vi "LSCE1.vi"(0 "时间间隔":dbl format="%#_13g", 3 "数值输入控件":i32, 4 "相关函数":cluster{"f0":dbl, "df":dbl, "magnitude":dbl[]}(graph), 5 "FRF Phase":cluster{"f0":dbl, "df":dbl, "magnitude":dbl[]}(graph), 6 "FRF magnifitude":cluster{"f0":dbl, "df":dbl, "magnitude":dbl[]}(graph)) -> (1 "模态阻尼比":dbl[](array[numeric]), 2 "模态频率":dbl[](array[numeric]))   [LabVIEW 2014]
uses:
  <vilib>/Analysis/2dsp.llb/Inverse Real FFT.vi
  <vilib>/Analysis/baseanly.llb/Real A x B.vi
  <vilib>/Analysis/baseanly.llb/A x Vector.vi
  <vilib>/Analysis/baseanly.llb/Real Inverse Matrix.vi
  <vilib>/Analysis/polynomials.llb/Polynomial Roots (DBL).vi
  <vilib>/Analysis/NI_AALPro.lvlib
  <vilib>/Analysis/NI_AALBase.lvlib
panel:
  in  "error out":errorcluster caption="错误输出"
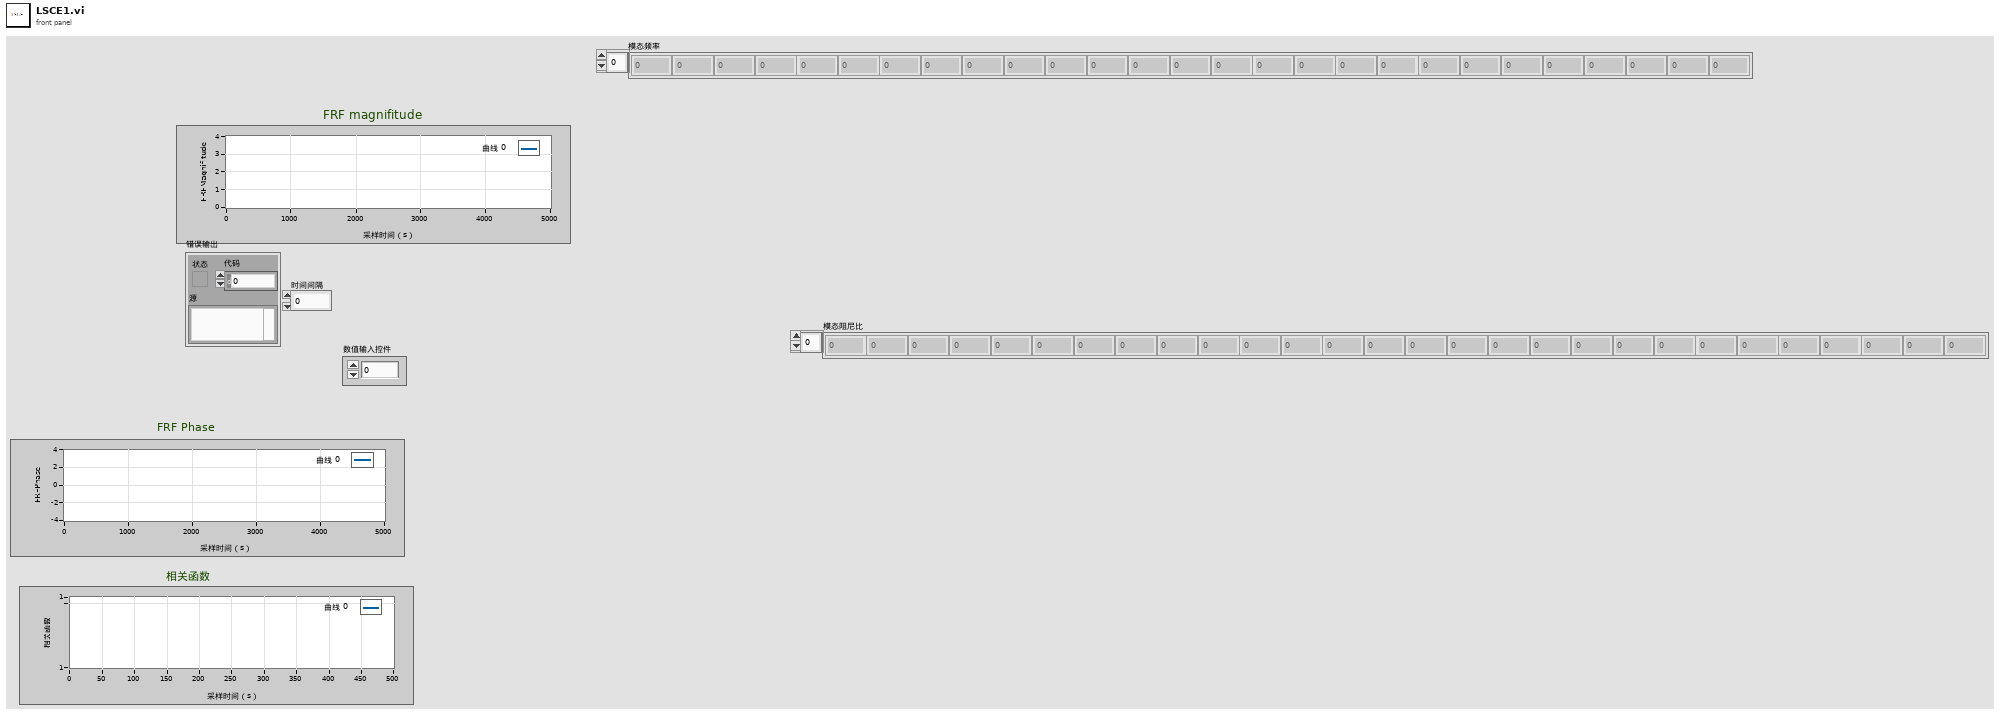
[diagram p1: front panel]
types:
  T1 = typedef "NI_Matrix.lvlib/RealMatrix.ctl" = dbl[][]
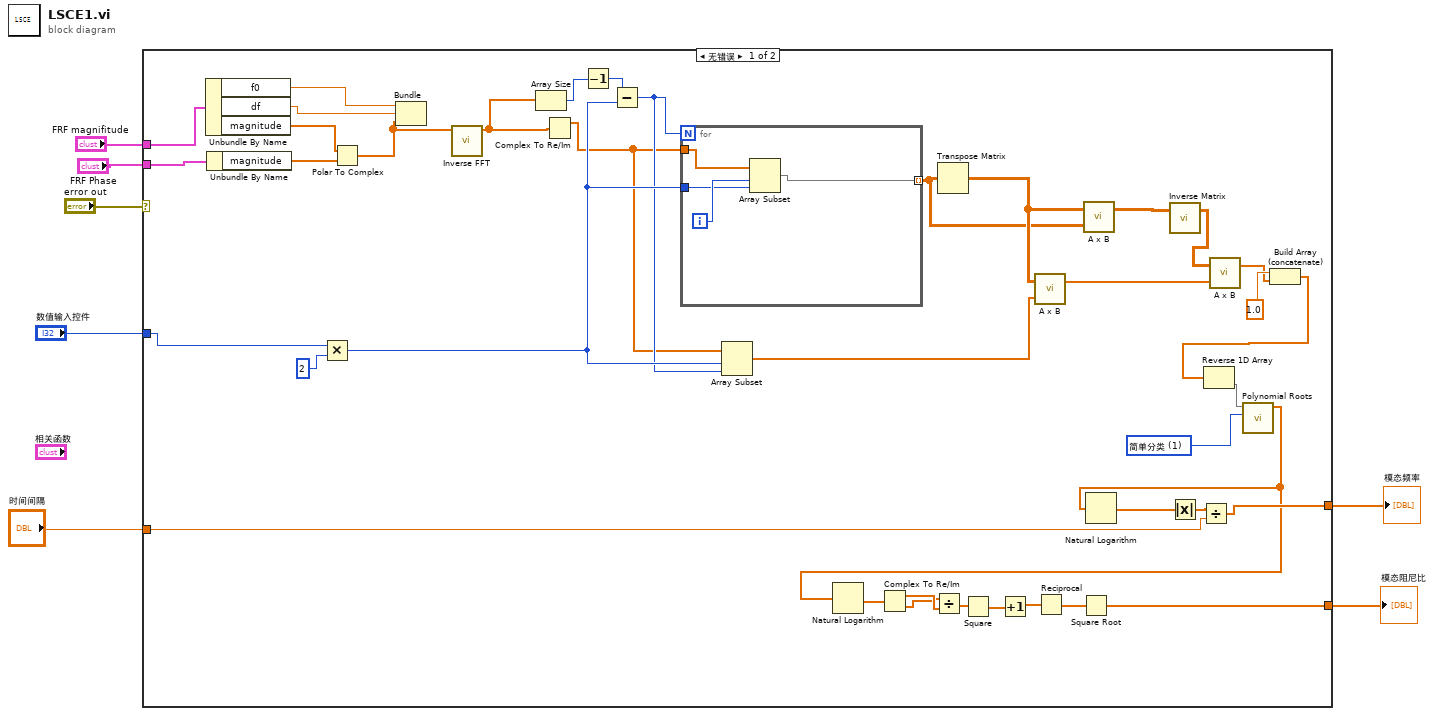
[diagram p0: block diagram]
diagram:
  n1 = case shown="无错误" "error out" {
    tunnel: "FRF magnifitude" -> [w46 _]
    tunnel: "FRF Phase" -> [w45 _]
    tunnel: "数值输入控件" -> [w39 _]
    tunnel: [w28 _] -> w3
    tunnel: [w20 _] -> w2
    tunnel: "时间间隔" -> [w8 _]
    frame No Error {
      w32 = u16 1 items=["常规", "简单分类", "精确", "高级精确"] ("option")
      n2 = Unbundle By Name(w46) -> ("f0"=w42:dbl, "df"=w29:dbl, "magnitude"=w44:dbl[])
      n3 = Unbundle By Name(w45) -> ("magnitude"=w43:dbl[])
      n4 = Multiply(x=w39, y=2) -> (x*y=w35:i32)
      n5 = Polar To Complex(1:w43, 2:w44) -> (0:w41:cdb[])
      n6 = Bundle("f0"=w42, "df"=w29, w41) -> ()  [unwired: 1 in, 1 out]
      n7 = call-poly <vilib>:"Inverse FFT.vi"("FFT {X}"=w41) -> ("X"=w40:dbl[])  [unwired: 9 in, 1 out]
      n8 = Array Size(array=w40) -> (size(s)=w37:i32)
      n9 = Complex To Re/Im(x + iy=w40) -> (x=w33:dbl[])  [unwired: 1 out]
      n10 = Decrement(x=w37) -> (x-1=w36:i32)
      n11 = Subtract(x=w36, y=w35) -> (x-y=w34:i32)
      n12 = for {
        N: w34 -> [_]
        tunnel: w33 -> [w50]
        tunnel: w35 -> [w48]
        tunnel: [w47] -> w13 mode=indexing
        i -> [w49]
        n13 = Array Subset(array=w50, index=w49, length=w48) -> (w47:dbl[])
      }
      n14 = Array Subset(array=w33, index=w35, length=w34) -> (w17:dbl[])
      n15 = Transpose Matrix(1:w13) -> (0:w14:dbl[][])
      n16 = call-poly <vilib>:"A x B.vi"("Vector"=w17, "A"=w14) -> ("A x Vector"=w16:dbl[])  [unwired: 1 out]
      n17 = call-poly <vilib>:"A x B.vi"("B"=w13, "A"=w14) -> ("A x B"=w15:T1)  [unwired: 1 out]
      n18 = call-poly <vilib>:"Inverse Matrix.vi"("Input Matrix"=w15) -> ("Inverse Matrix"=w18:T1)  [unwired: 1 in, 1 out]
      n19 = call-poly <vilib>:"A x B.vi"("Vector"=w16, "A"=w18) -> ("A x Vector"=w9:dbl[])  [unwired: 1 out]
      n20 = Build Array (concatenate)(1.0, w9) -> (w12:dbl[])
      n21 = Reverse 1D Array(array=w12) -> (reversed array=w19:dbl[])
      n22 = call-poly <vilib>:"Polynomial Roots.vi"("option"=w32, "P(x)"=w19) -> ("Roots"=w11:cdb[])  [unwired: 8 in, 1 out]
      n23 = Natural Logarithm(1:w11) -> (0:w27:cdb[])
      n24 = Complex To Re/Im(x + iy=w27) -> (x=w26:dbl[], y=w25:dbl[])
      n25 = Divide(x=w25, y=w26) -> (x/y=w24:dbl[])
      n26 = Square(x=w24) -> (x^2=w23:dbl[])
      n27 = Increment(x=w23) -> (x+1=w22:dbl[])
      n28 = Reciprocal(x=w22) -> (1/x=w21:dbl[])
      n29 = Square Root(x=w21) -> (sqrt(x)=w20:dbl[])
      n30 = Natural Logarithm(1:w11) -> (0:w31:cdb[])
      n31 = Absolute Value(x=w31) -> (abs(x)=w30:dbl[])
      n32 = Divide(x=w30, y=w8) -> (x/y=w28:dbl[])
    }
    frame Error {
    }
  }
  "模态频率" <- w3
  "模态阻尼比" <- w2
